vi "数据查询_数据查询.vi"() -> ()   [LabVIEW 2016]
uses:
  <vilib>/Utility/miscctls.llb/LVPointTypeDef.ctl
  <vilib>/Utility/miscctls.llb/LVRowAndColumnUnsignedTypeDef.ctl
  <userlib>/_OpenG.lib/array/array.llb/Sort 2D Array (String)__ogtk.vi
  <vilib>/addons/database/_DB Variant To Data/Database Variant To Data.xnode
panel:
  in  "下拉列表":string(xcontrol)
  in  "导出":bool
  out "分钟小时":string(combo)="实时数据"
  out "工作类型":string(combo)="全部数据"
  out "连接的字符串":string
  out "选中数据表":string
  in  "查询":bool
  in  "结束日期":string="2050/01/01"
  in  "起始日期":string="2010/01/01"
  out "XY图":cluster{"data":timestamp[], "data":dbl[]}[](graph)
  out "数据表":string[][](table)
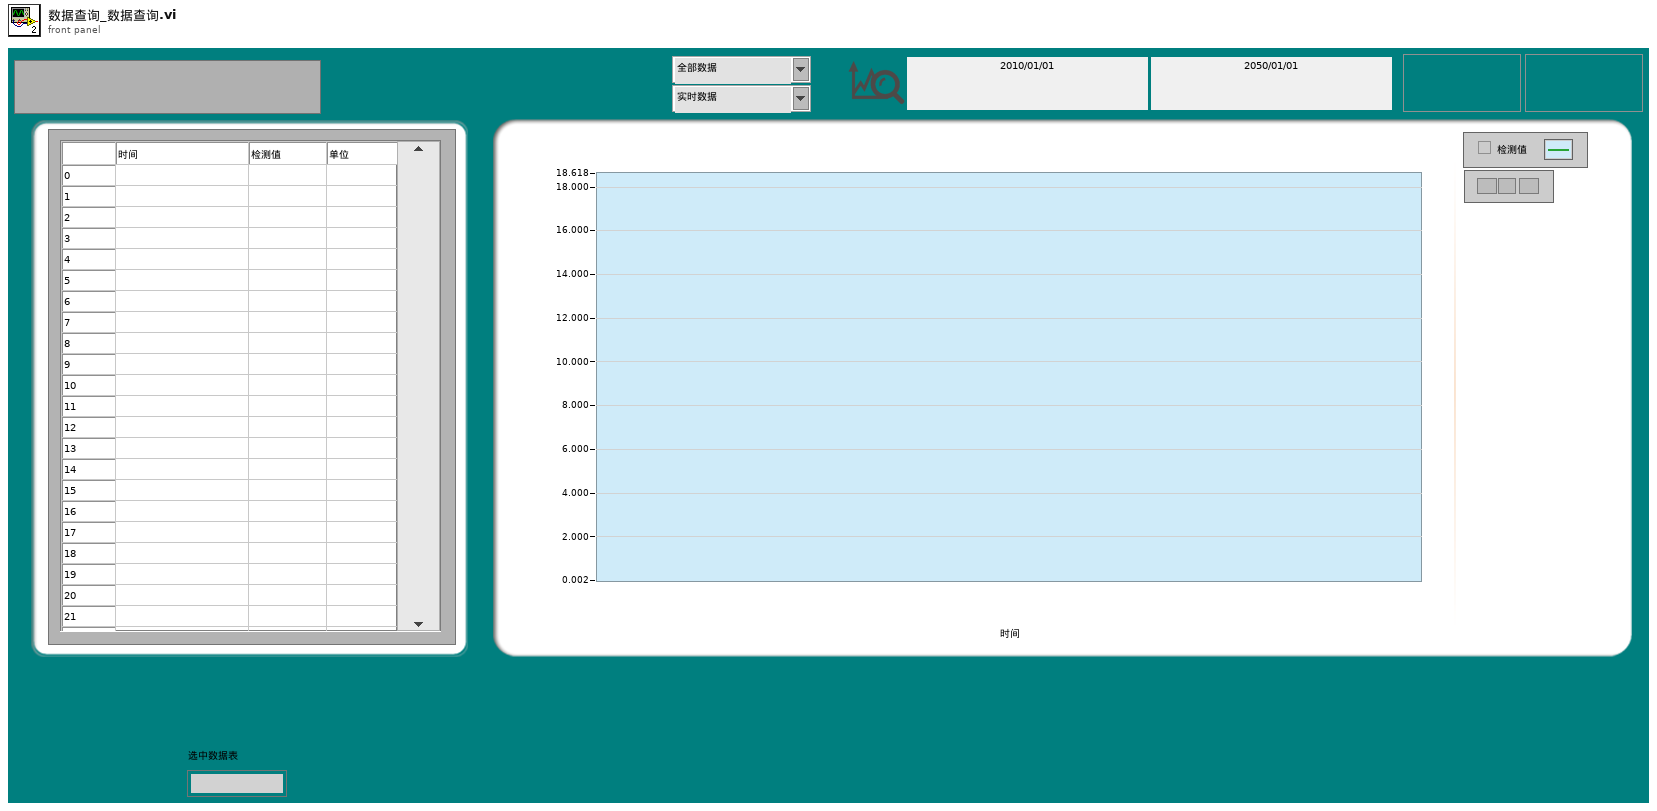
[diagram p1: front panel]
types:
  T1 = typedef "LVPointTypeDef.ctl" = cluster{"Horizontal":i16, "Vertical":i16}
  T2 = enum8{"Enabled", "Disabled", "Disabled and Grayed Out"}
  T3 = typedef "LVRowAndColumnUnsignedTypeDef.ctl" = cluster{"Row":u32, "Column":u32}
  T4 = typedef "LVPoint32TypeDef.ctl" = cluster{"Horizontal":i32, "Vertical":i32}
  T5 = typedef "LVPointDoubleTypeDef.ctl" = cluster{"Cursor X":dbl, "Cursor Y":dbl}
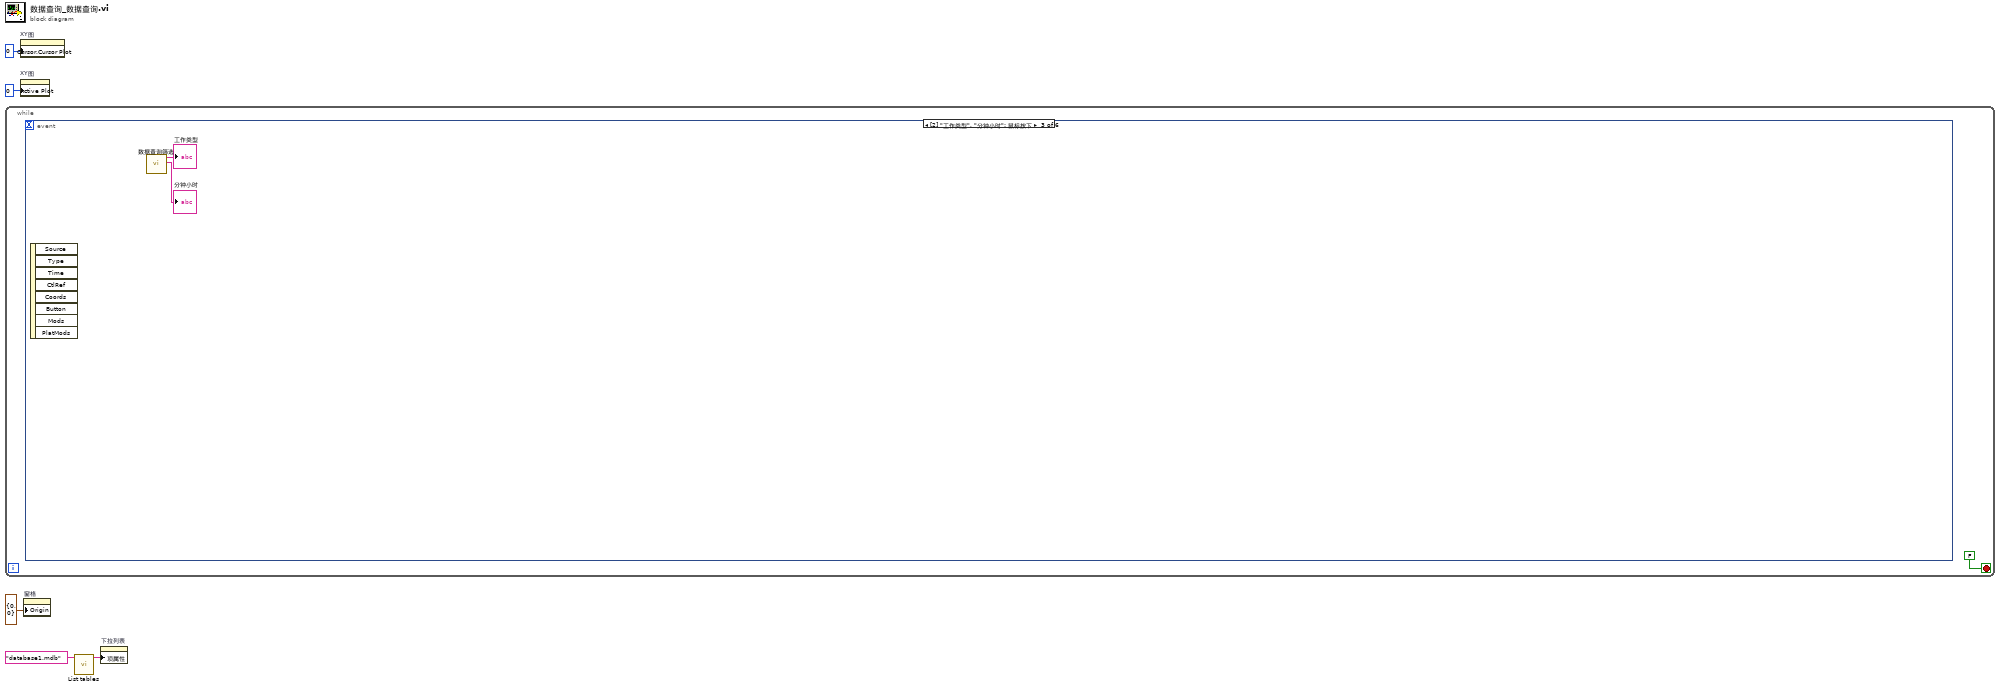
[diagram p0: block diagram]
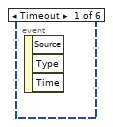
[diagram p2: hidden frame]
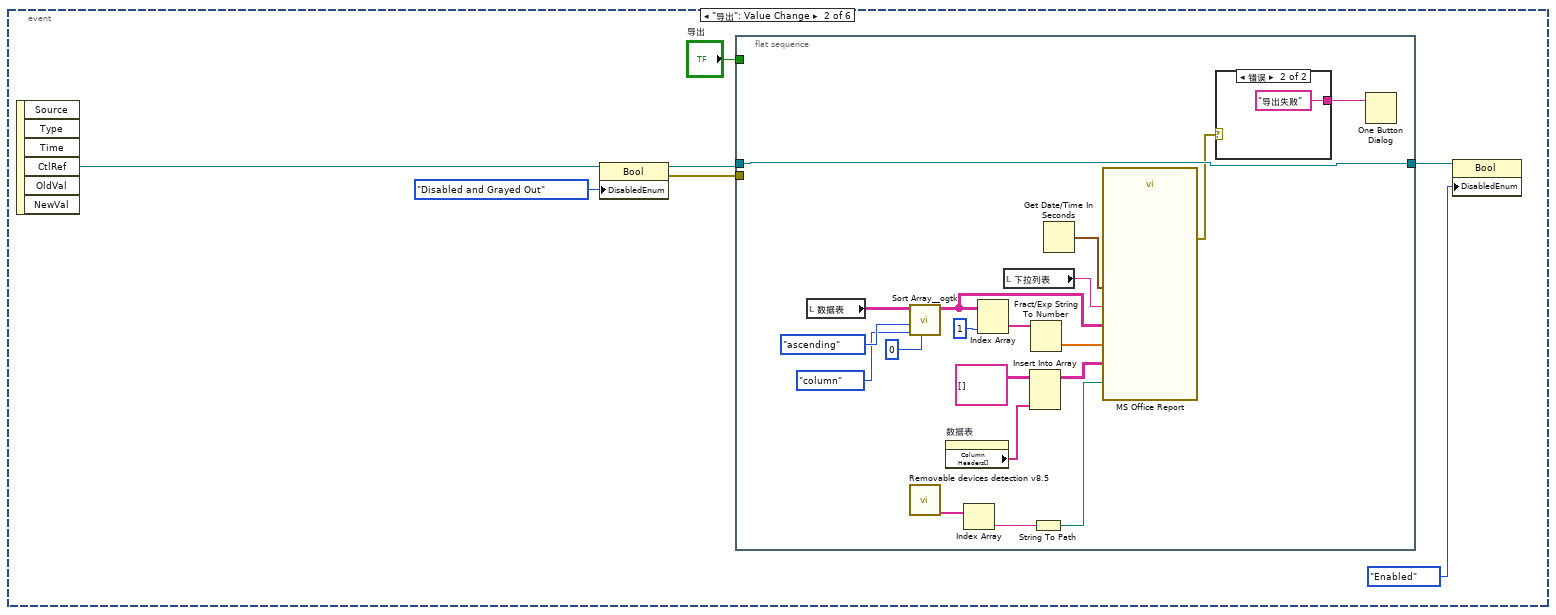
[diagram p3: hidden frame]
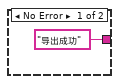
[diagram p4: hidden frame]
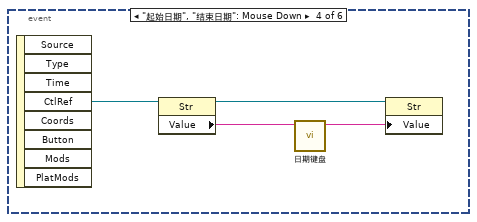
[diagram p5: hidden frame]
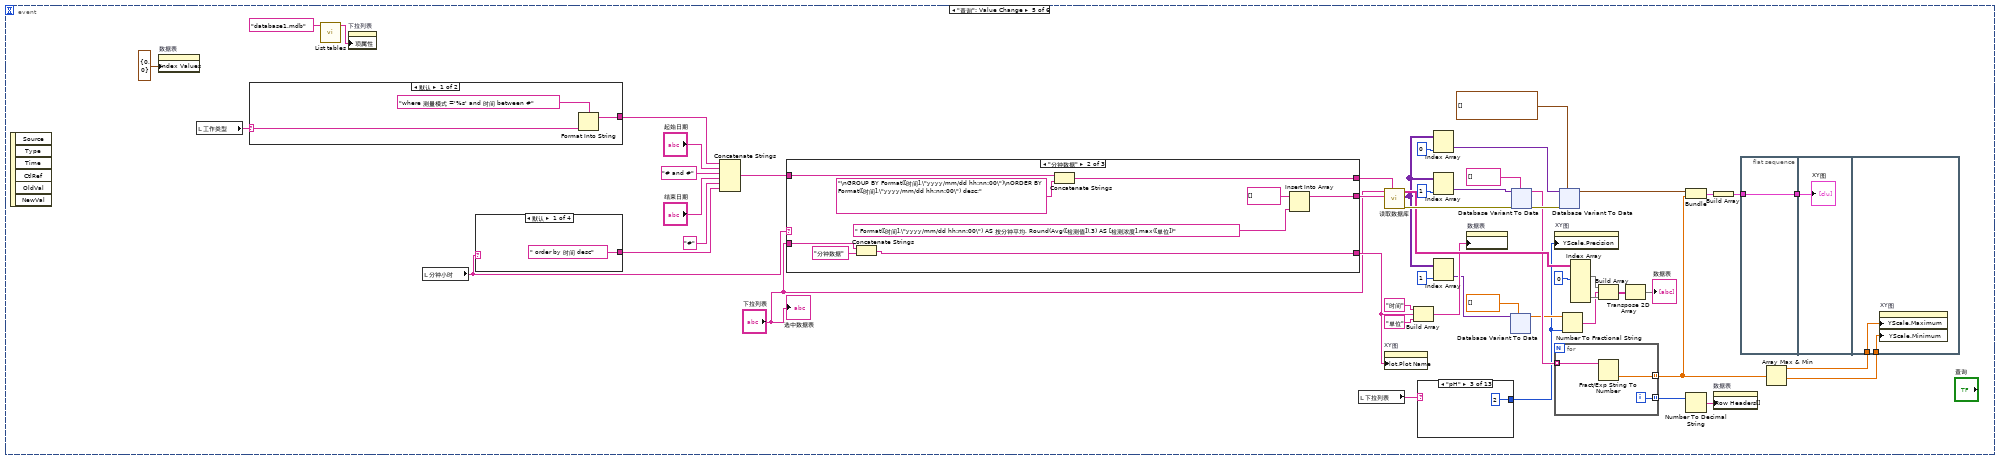
[diagram p6: hidden frame]
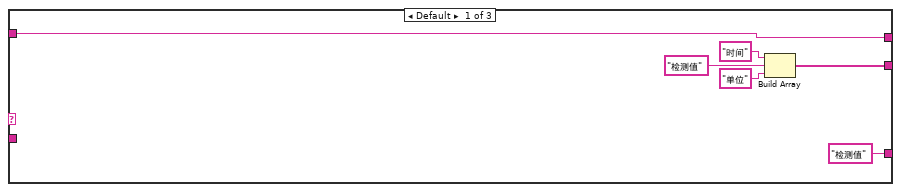
[diagram p7: hidden frame]
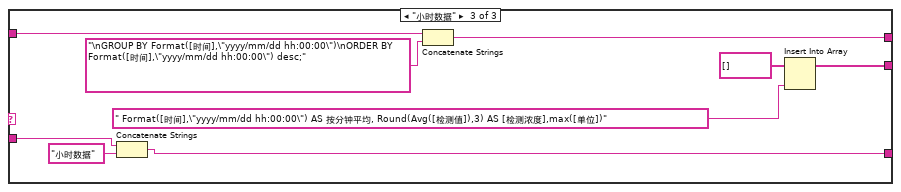
[diagram p8: hidden frame]
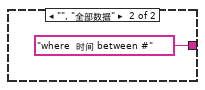
[diagram p12: hidden frame]
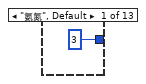
[diagram p13: hidden frame]
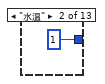
[diagram p14: hidden frame]
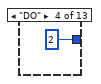
[diagram p15: hidden frame]
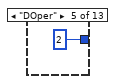
[diagram p16: hidden frame]
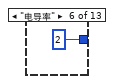
[diagram p17: hidden frame]
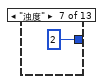
[diagram p18: hidden frame]
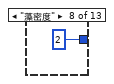
[diagram p19: hidden frame]
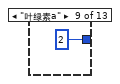
[diagram p20: hidden frame]
diagram:
  n1 = while {
    stop <- FALSE stop-if-true
    n2 = event shown="[2] \"工作类型\", \"分钟小时\": 鼠标按下" {
      selector: _ -> [_ _ _ _ _ _]
      dyn-events: _ -> [_ _ _ _ _ _]
      timeout: _ -> [_ _ _ _ _ _]
      event Timeout {
        n3 = event-data() -> ()  [unwired: 1 in, 3 out]
      }
      event "导出": Value Change {
        n4 = event-data() -> ("CtlRef"=w13:refnum<vi>)  [unwired: 1 in, 5 out]
        n5 = property class="Bool"(reference=w13, "DisabledEnum"=T2."Disabled and Grayed Out" ("禁用")) -> (reference out=w10:refnum<vi>, error out=w11:errorcluster)  [unwired: 1 in]
        n6 = flat-sequence {
          tunnel: w11 -> [_]
          tunnel: [w22] -> w9
          tunnel: w10 -> [w22]
          tunnel: "导出" -> [_]
          frame #0 {
            n7 = local read "数据表"() -> (w30:string[][])
            n8 = call-poly <userlib>:"Sort Array__ogtk.vi"("Column/Row to Sort By"=u32 0, "Sort By in"=enum16{"row", "column"}."column", "Order"=enum16{"ascending", "descending"}."ascending", "Array in"=w30) -> ("Sorted Array out"=w29:string[][])  [unwired: 4 in, 3 out]
            n9 = call "Removable devices detection v8.5.vi"() -> ("Removable"=w19:string[])  [unwired: 4 out]
            n10 = property on="数据表" class="Tbl (严格)"() -> ("Column Headers[]"=w15:string[])  [unwired: 2 in, 2 out]
            n11 = Index Array(array=w19) -> (element=w18:string)  [unwired: 1 in]
            n12 = Index Array(array=w29, index (col)=1 ("禁用的索引 (列)")) -> (element=w25:string[])  [unwired: 1 in]
            n13 = local read "下拉列表"() -> (w23:string)
            n14 = Insert Into Array(array=string[][] [], new element=w15) -> (w14:string[][])  [unwired: 2 in]
            n15 = Fract/Exp String To Number(string=w25) -> (number=w24:dbl[])  [unwired: 3 in, 1 out]
            n16 = String To Path(string=w18) -> (path=w17:path)
            n17 = Get Date/Time In Seconds() -> (seconds since 1Jan1904=w32:timestamp)
            n18 = call "MS Office Report"("Path to Save Report"=w17, "导出日期"=w32, "监测参数"=w23, "数据输入"=w29, "图表输入"=w24, "字段定义"=w14) -> ("error out"=w21:errorcluster)  [unwired: 20 in, 1 out]
            n19 = case shown="错误" w21 {
              tunnel: ["导出成功" ("消息") "导出失败" ("消息")] -> w20
              frame No Error {
              }
              frame Error {
              }
            }
            n20 = One Button Dialog(message=w20) -> ()  [unwired: 1 in, 1 out]
          }
        }
        n21 = property class="Bool"(reference=w9, "DisabledEnum"=T2."Enabled" ("禁用")) -> ()  [unwired: 1 in, 2 out]
      }
      event "工作类型", "分钟小时": Mouse Down {
        n22 = event-data() -> ()  [unwired: 1 in, 8 out]
        n23 = call "数据查询筛选.vi"() -> ("分钟小时"=→"分钟小时":string, "工作类型"=→"工作类型":string)  [unwired: 10 in]
      }
      event "起始日期", "结束日期": Mouse Down {
        n24 = event-data() -> ("CtlRef"=w40:refnum<vi>)  [unwired: 1 in, 7 out]
        n25 = property class="Str"(reference=w40) -> (reference out=w38:refnum<vi>, "Value"=w39:string)  [unwired: 1 in, 1 out]
        n26 = call "日期键盘.vi"("原值"=w39) -> ("x+y"=w37:string)  [unwired: 10 in]
        n27 = property class="Str"(reference=w38, "Value"=w37) -> ()  [unwired: 1 in, 2 out]
      }
      event "查询": Value Change {
        n28 = event-data() -> ()  [unwired: 1 in, 6 out]
        n29 = property on="数据表" class="Tbl (严格)"("Index Values"=T3 {"Row"=0, "Column"=0} ("索引值")) -> ()  [unwired: 2 in, 2 out]
        n30 = local read "工作类型"() -> (w52:string)
        n31 = case shown="默认" w52 {
          selector: w52 -> [w119 _]
          tunnel: [w117 "where  时间 between #" ("condition")] -> w51
          frame Default {
            n32 = Format Into String(format string="where 测量模式 ='%s' and 时间 between #" ("condition"), w119) -> (resulting string=w117:string)  [unwired: 2 in, 1 out]
          }
          frame "", "全部数据" {
          }
        }
        n33 = call "List tables.vi"("database"="database1.mdb") -> ("tables"=w41:string[])  [unwired: 9 in, 1 out]
        n34 = property on="下拉列表" class="下拉列表 (严格)"("项属性"=w41) -> ()  [unwired: 2 in, 2 out]
        n35 = local read "分钟小时"() -> (w48:string)
        n36 = case shown="默认" w48 {
          tunnel: [" order by 时间 desc" ("字符串") _ _ _] -> w50
          frame Default {
          }
          frame "分钟数据" {
          }
          frame "小时数据" {
          }
          frame "真" {
          }
        }
        n37 = Concatenate Strings(w51, "起始日期", "# and #" ("condition"), "结束日期", "#" ("condition"), w50) -> (w49:string)
        n38 = case shown="\"分钟数据\"" w48 {
          tunnel: [w93 w105 w110] -> w46
          tunnel: w49 -> [w97 w103 w112]
          tunnel: [w97 w102 w111] -> w47
          tunnel: ["检测值" w98 w107] -> w45
          tunnel: "下拉列表" -> [_ w99 w109]
          frame Default {
            n39 = Build Array("时间", "检测值", "单位" ("元素")) -> (w93:string[])
          }
          frame "分钟数据" {
            n40 = Concatenate Strings(w99, "分钟数据" ("字符串")) -> (w98:string)
            n41 = Concatenate Strings(w103, "\nGROUP BY Format([时间],\"yyyy/mm/dd hh:nn:00\")\nORDER BY Format([时间],\"yyyy/mm/dd hh:nn:00\") desc;" ("字符串")) -> (w102:string)
            n42 = Insert Into Array(array=string[] [] ("显示项"), new element=" Format([时间],\"yyyy/mm/dd hh:nn:00\") AS 按分钟平均, Round(Avg([检测值]),3) AS [检测浓度],max([单位])" ("新元素/子数组")) -> (w105:string[])  [unwired: 1 in]
          }
          frame "小时数据" {
            n43 = Concatenate Strings(w109, "小时数据" ("字符串")) -> (w107:string)
            n44 = Concatenate Strings(w112, "\nGROUP BY Format([时间],\"yyyy/mm/dd hh:00:00\")\nORDER BY Format([时间],\"yyyy/mm/dd hh:00:00\") desc;" ("字符串")) -> (w111:string)
            n45 = Insert Into Array(array=string[] [] ("显示项"), new element=" Format([时间],\"yyyy/mm/dd hh:00:00\") AS 按分钟平均, Round(Avg([检测值]),3) AS [检测浓度],max([单位])" ("新元素/子数组")) -> (w110:string[])  [unwired: 1 in]
          }
        }
        n46 = local read "下拉列表"() -> (w58:string)
        n47 = call "读取数据库.vi"("condition"=w47, "显示项"=w46, "组合框"="下拉列表") -> ("error out"=w82:errorcluster, "data"=w65:variant[][], "表格"=w75:string[][])  [unwired: 5 in, 1 out]
        n48 = property on="XY图" class="XYGraph (严格)"("Plot.Plot Name"=w45) -> ()  [unwired: 2 in, 2 out]
        n49 = Build Array("时间", w45, "单位" ("元素")) -> (w69:string[])
        n50 = case shown="\"pH\"" w58 {
          tunnel: [i16 3 ("精度(6)") i16 1 ("精度(6)") i16 2 ("精度(6)") i16 2 ("精度(6)") i16 2 ("精度(6)") i16 2 ("精度(6)") i16 2 ("精度(6)") i16 2 ("精度(6)") i16 2 ("精度(6)") i16 3 ("精度(6)") i16 2 ("精度(6)") i16 2 ("精度(6)") i16 2 ("精度(6)")] -> w53
          frame "氨氮", Default {
          }
          frame "水温" {
          }
          frame "pH" {
          }
          frame "DO" {
          }
          frame "DOper" {
          }
          frame "电导率" {
          }
          frame "浊度" {
          }
          frame "藻密度" {
          }
          frame "叶绿素a" {
          }
          frame "总磷" {
          }
          frame "总氮" {
          }
          frame "CodCr" {
          }
          frame "CodMn" {
          }
        }
        n51 = Index Array(array=w65, index (col)=0 ("禁用的索引 (列)")) -> (element=w85:variant[])  [unwired: 1 in]
        n52 = Index Array(array=w65, index (col)=1 ("禁用的索引 (列)")) -> (element=w83:variant[])  [unwired: 1 in]
        n53 = Index Array(array=w65, index (col)=1 ("禁用的索引 (列)")) -> (element=w63:variant[])  [unwired: 1 in]
        n54 = property on="数据表" class="Tbl (严格)"("Column Headers[]"=w69) -> ()  [unwired: 2 in, 2 out]
        n55 = xnode "Database Variant To Data"("database variant"=w63, "type"=sgl[] []) -> ("data"=w61:sgl[])  [unwired: 1 in, 1 out]
        n56 = xnode "Database Variant To Data"("database variant"=w83, "error in (no error)"=w82, "type"=string[] []) -> ("data"=w68:string[], "error out"=w81:errorcluster)
        n57 = property on="XY图" class="XYGraph (严格)"("YScale.Precision"=w53) -> ()  [unwired: 2 in, 2 out]
        n58 = for {
          tunnel: w68 -> [w174] mode=indexing
          tunnel: [w173] -> w56 mode=indexing
          tunnel: [w172] -> w44 mode=indexing
          i -> [w172]
          n59 = Fract/Exp String To Number(string=w174) -> (number=w173:dbl)  [unwired: 3 in, 1 out]
        }
        n60 = xnode "Database Variant To Data"("database variant"=w85, "error in (no error)"=w81, "type"=timestamp[] []) -> ("data"=w76:timestamp[])  [unwired: 1 out]
        n61 = Number To Fractional String(number=w61, precision (6)=w53) -> (F-format string=w60:string[])  [unwired: 2 in]
        n62 = Index Array(array=w75, index (col) #1=0 ("禁用的索引 (列)")) -> (element #1=w73:string[], element #3=w66:string[])  [unwired: 5 in, 1 out]
        n63 = Build Array(w73, w60, w66) -> (w72:string[][])
        n64 = Transpose 2D Array(2D array=w72) -> (transposed array=→"数据表":string[][])
        n65 = Bundle("data"=w76, w56) -> (w77:cluster{"data":timestamp[], dbl[]})  [unwired: 1 in]
        n66 = Number To Decimal String(number=w44) -> (decimal integer string=w43:string[])  [unwired: 1 in]
        n67 = Build Array(w77) -> (w78:cluster{"data":timestamp[], dbl[]}[])
        n68 = property on="数据表" class="Tbl (严格)"("Row Headers[]"=w43) -> ()  [unwired: 2 in, 2 out]
        n69 = flat-sequence {
          tunnel: [w175] -> w79
          tunnel: w78 -> [w175]
          tunnel: w79 -> [w176]
          tunnel: w55 -> [w178]
          tunnel: w54 -> [w177]
          frame #0 {
          }
          frame #1 {
            "XY图" <- w176
          }
          frame #2 {
            n70 = property on="XY图" class="XYGraph (严格)"("YScale.Maximum"=w178, "YScale.Minimum"=w177) -> ()  [unwired: 2 in, 2 out]
          }
        }
        n71 = Array Max & Min(array=w56) -> (max value=w55:dbl, min value=w54:dbl)  [unwired: 2 out]
        "选中数据表" <- "下拉列表"
      }
      event "XY图": Mouse Move {
        w273 = "   " ("字符串")
        n72 = event-data() -> ("CtlRef"=w283:refnum<vi>, "Coords"=w282:T4)  [unwired: 1 in, 3 out]
        n73 = invoke class="XYGraph (严格)" method="Map Coords To XY"(reference=w283, "Coords"=w282) -> (reference out=w281:refnum<vi>, error out=w278:errorcluster, "XY"=w280:cluster{"X":dbl, "Y":dbl})  [unwired: 5 in, 4 out]
        n74 = property class="XYGraph (严格)"(reference=w281, error in=w278, "Cursor.Cursor Position"=w280) -> (error out=w279:errorcluster)  [unwired: 1 out]
        n75 = property on="XY图" class="XYGraph (严格)"(error in=w279) -> ("Cursor.Cursor Position"=w276:T5, "YScale.Precision"=w269:u8)  [unwired: 1 in, 2 out]
        n76 = Unbundle(w276) -> ("Cursor X"=w275:dbl, "Cursor Y"=w272:dbl)
        n77 = property on="XY图" class="XYGraph (严格)"() -> ("Plot.Plot Name"=w270:string)  [unwired: 2 in, 2 out]
        n78 = Number To Fractional String(number=w272, precision (6)=w269) -> (F-format string=w271:string)  [unwired: 2 in]
        n79 = Format Date/Time String(seconds (now)=w275) -> (date/time string=w274:string)  [unwired: 2 in]
        n80 = Concatenate Strings(w270, w273, w274, w273, w271) -> (→"连接的字符串":string)
      }
    }
  }
  n81 = property on="XY图" class="XYGraph (严格)"("Cursor.Cursor Plot"=0 ("游标.游标关联曲线")) -> ()  [unwired: 2 in, 2 out]
  n82 = property on="XY图" class="XYGraph (严格)"("Active Plot"=u32 0 ("活动曲线")) -> ()  [unwired: 2 in, 2 out]
  n83 = property on="窗格" class="Pane"("Origin"=T1 {"Horizontal"=0, "Vertical"=0} ("原点")) -> ()  [unwired: 2 in, 2 out]
  n84 = call "List tables.vi"("database"="database1.mdb") -> ("tables"=w1:string[])  [unwired: 9 in, 1 out]
  n85 = property on="下拉列表" class="下拉列表 (严格)"("项属性"=w1) -> ()  [unwired: 2 in, 2 out]
